vi "MSFET202_Input&Output.vi"(0 "Data Saved":path=path "C:/Users/Garrett/Google Drive/Documents/Martz Lab/MSFET/Raw Data & Matlab/pH_Voltages208.csv", 1 "Sensor":string(combo)="MSFET 208", 3 "Boolean":bool, 4 "Weighting (Sample)":enum16{"Sample", "Population"}(ring), 5 "Temp Voltage":dbl[](array[numeric])=[0.8626518823444147, 0.8626518823444147, 0.8626518823444147, 0.8628162805593685, 0.8629806787744291, 0.8626518823444147, 0.8624874841295675, 0.8631450769895964, 0.8628162805593685, 0.8629806787744291] format="%0.2f", 6 "ISFET Voltage\\":dbl[](array[numeric])=[0.9538929084585316, 0.9535641119060577, 0.9540573067349407, 0.9543861032881034, 0.9535641119060577, 0.9538929084585316, 0.9537285101822373, 0.954550501564857, 0.9542217050114647, 0.954550501564857], 7 "REF Voltage":dbl[](array[numeric])=[0.5945185251348065, 0.5941897290141942, 0.5940253309540122, 0.5940253309540122, 0.5941897290141942, 0.593860932893913, 0.594354127074459, 0.594354127074459, 0.5941897290141942, 0.594354127074459], 8 "DirecTemp":dbl=23.4) -> (12 "Temperature (C)":dbl=22.076639633423227, 13 "Mean1":dbl=0.9540408669075637 format="%.5f", 14 "std0":dbl=0.00018672030324610737 format="%.6f", 15 "Mean0":dbl=0.5942061688202704 format="%.6f", 18 "std1":dbl=0.0003560276121429779 format="%.5f", 19 "pHint":dbl=8.584275147135203)   [LabVIEW 2018]
uses:
  <vilib>/Utility/file.llb/Write Delimited Spreadsheet (string).vi
  <vilib>/Analysis/NI_AALBase.lvlib
panel:
  out "Waveform Graph":dbl[](graph)
  out "std1 2":dbl=0.00020209022026499576 format="%.5f"
  out "Mean1 2":dbl=0.8627834009164419 format="%.5f"
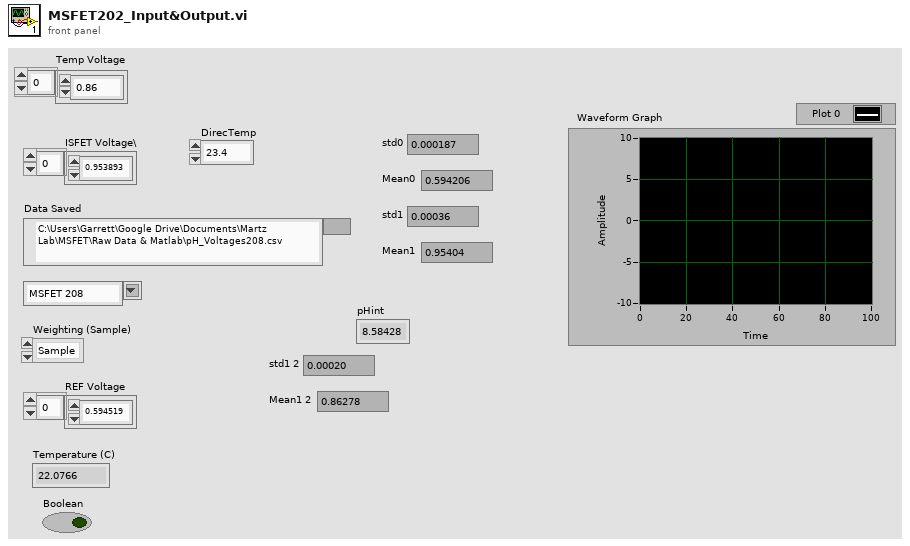
[diagram p1: front panel]
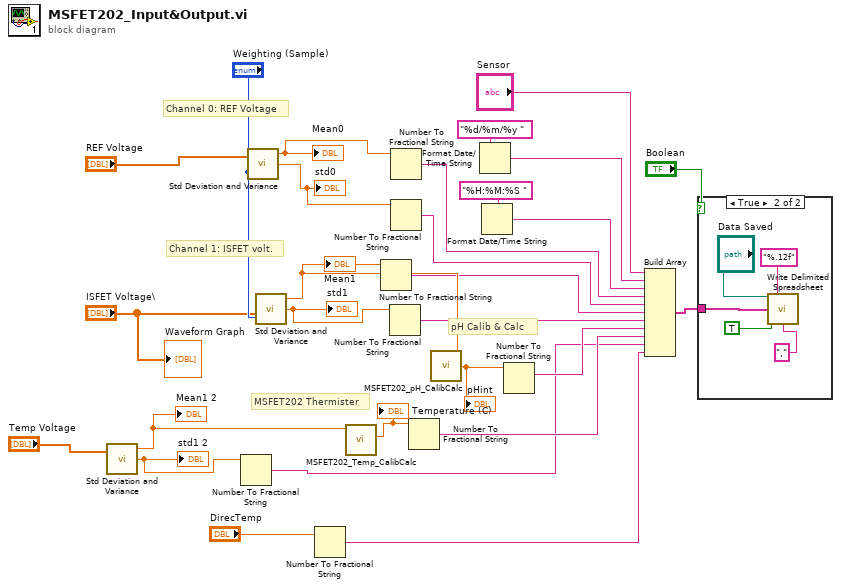
[diagram p0: block diagram]
diagram:
  # "MSFET202 Thermister"
  # "Channel 0: REF Voltage"
  # "Channel 1: ISFET volt."
  # "pH Calib & Calc"
  n1 = call <vilib>:"Std Deviation and Variance.vi"("X"="Temp Voltage") -> ("mean"=w5:dbl, "standard deviation"=w10:dbl)  [unwired: 1 in, 1 out]
  "Mean1 2" <- w5
  "std1 2" <- w10
  n2 = Number To Fractional String(number=w10) -> (F-format string=w7:string)  [unwired: 3 in]
  n3 = call <vilib>:"Std Deviation and Variance.vi"("X"="REF Voltage", "Weighting (Sample)"="Weighting (Sample)") -> ("mean"=w18:dbl, "standard deviation"=w23:dbl)  [unwired: 1 out]
  "Mean0" <- w18
  "std0" <- w23
  n4 = call <vilib>:"Std Deviation and Variance.vi"("X"="ISFET Voltage\\", "Weighting (Sample)"="Weighting (Sample)") -> ("mean"=w22:dbl, "standard deviation"=w17:dbl)  [unwired: 1 out]
  "Mean1" <- w22
  "std1" <- w17
  n5 = Number To Fractional String(number="DirecTemp") -> (F-format string=w2:string)  [unwired: 3 in]
  n6 = call "MSFET202_Temp_CalibCalc.vi"("\"VTherm\""=w5) -> ("Temperature (C)"=w6:dbl)  [unwired: 10 in]
  "Temperature (C)" <- w6
  n7 = Number To Fractional String(number=w22) -> (F-format string=w11:string)  [unwired: 3 in]
  n8 = Number To Fractional String(number=w17) -> (F-format string=w20:string)  [unwired: 3 in]
  n9 = Number To Fractional String(number=w18) -> (F-format string=w25:string)  [unwired: 3 in]
  n10 = Number To Fractional String(number=w23) -> (F-format string=w24:string)  [unwired: 3 in]
  n11 = Number To Fractional String(number=w6) -> (F-format string=w9:string)  [unwired: 3 in]
  n12 = call "MSFET202_pH_CalibCalc.vi"("Eint"=w22) -> ("pHint"=w21:dbl)
  "pHint" <- w21
  n13 = Format Date/Time String(time format string (%c)="%d/%m/%y ") -> (date/time string=w27:string)  [unwired: 2 in]
  n14 = Format Date/Time String(time format string (%c)="%H:%M:%S ") -> (date/time string=w28:string)  [unwired: 2 in]
  n15 = Number To Fractional String(number=w21) -> (F-format string=w19:string)  [unwired: 3 in]
  n16 = Build Array("Sensor", w27, w28, w25, w24, w11, w20, w19, w9, w7, w2) -> (w14:string[])
  n17 = case shown="True" "Boolean" {
    tunnel: w14 -> [_ w29]
    frame False {
    }
    frame True {
      n18 = call-poly <vilib>:"Write Delimited Spreadsheet.vi"("file path (dialog if empty)"="Data Saved", "format (%s)"="%.12f" ("format (%.3f)"), "1D data"=w29, "append to file? (new file:F)"=TRUE, "delimiter (\\t)"="," ("delimiter (\\t)")) -> ()  [unwired: 9 in, 2 out]
    }
  }
  "Waveform Graph" <- "ISFET Voltage\\"
